vi "取值范围-年月日下拉取值范围.vi"(8 "最小日期":i32[](array[numeric]), 9 "日":refnum<vi>, 10 "月":refnum<vi>, 11 "年":refnum<vi>) -> (0 "错误输出":errorcluster)   [LabVIEW 2017]
uses:
  <vilib>/Utility/miscctls.llb/LVStringsAndValuesArrayTypeDef_U16.ctl
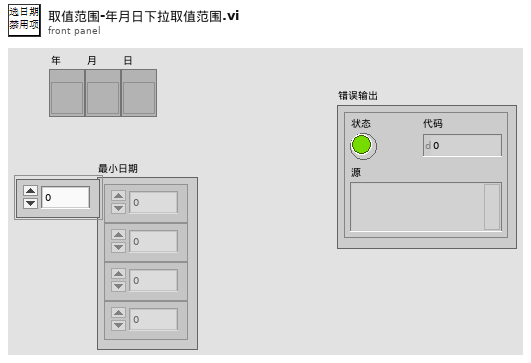
[diagram p1: front panel]
types:
  T1 = typedef "LVStringsAndValuesArrayTypeDef_U16.ctl" = cluster{"String":string, "Value":u16}[]
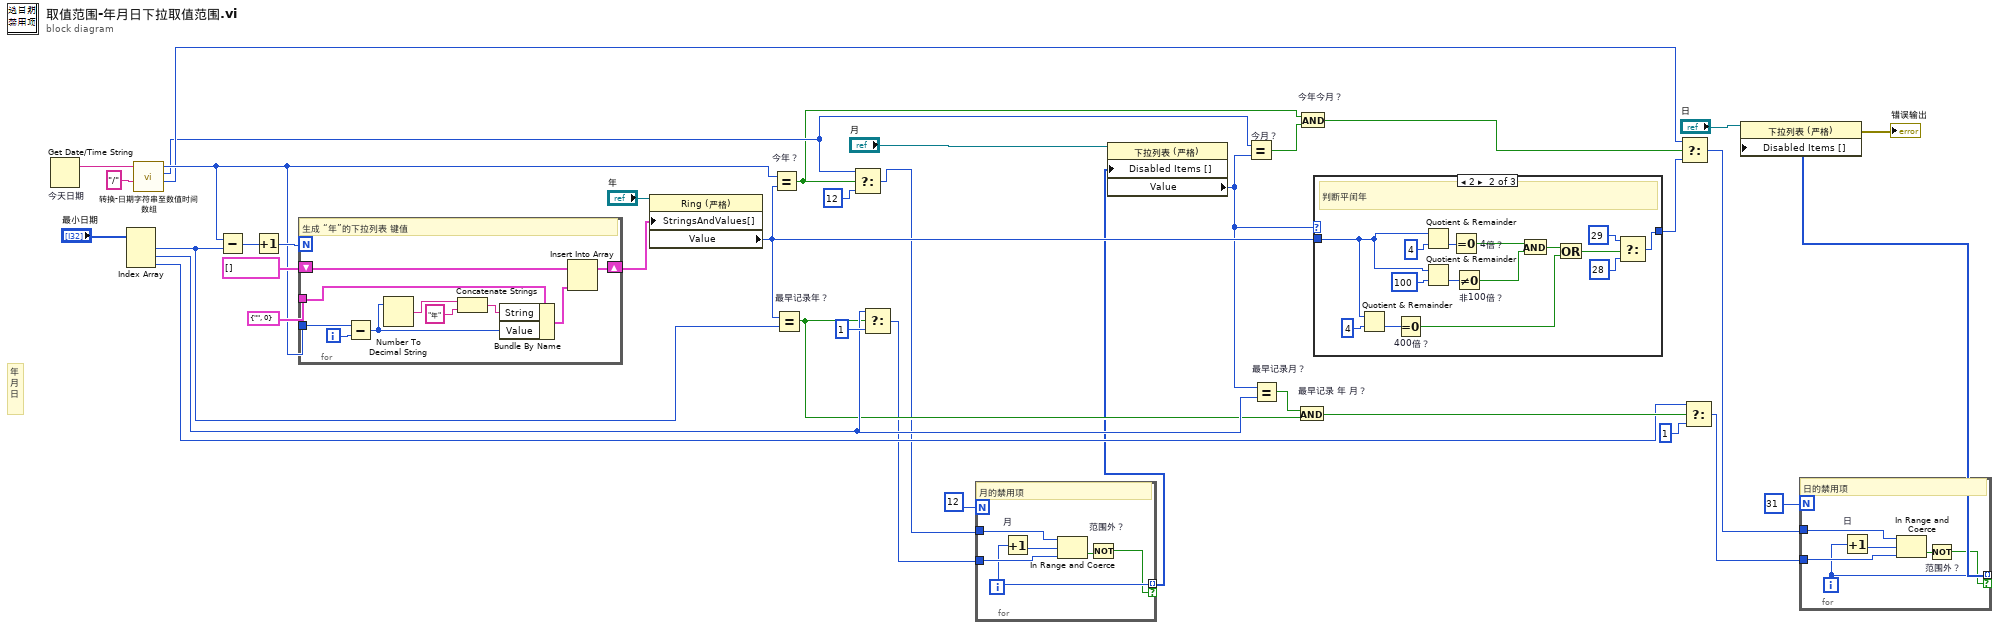
[diagram p0: block diagram]
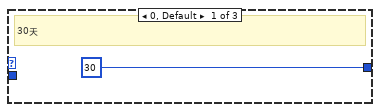
[diagram p2: hidden frame]
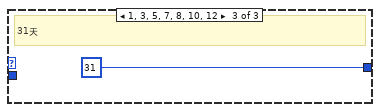
[diagram p3: hidden frame]
diagram:
  # "年\n月\n日"
  n1 = Get Date/Time String "今天日期"() -> (date string=w38:string)  [unwired: 3 in, 1 out]
  n2 = Index Array(array="最小日期") -> (element #1=w21:i32, element #2=w19:i32, element #3=w11:i32)  [unwired: 3 in]
  n3 = call "转换-日期字符串至数值时间数组.vi"("分隔符（/）"="/", "日期时间（或仅日期）字符串"=w38) -> ("D"=w25:i32, "M"=w24:i32, "Y"=w29:i32)  [unwired: 5 in, 2 out]
  n4 = Subtract(x=w29, y=w21) -> (x-y=w34:i32)
  n5 = Increment(x=w34) -> (x+1=w33:i32)
  n6 = for {
    N: w33 -> [_]
    tunnel: w29 -> [w48]
    shift-right: [w43] -> w30
    shift-left: T1 [] ("字符串与值[]") -> [w44]
    tunnel: cluster{"String":string, "Value":u16} {"String"="", "Value"=0} -> [w42]
    i -> [w47]
    # "生成 “年”的下拉列表 键值"
    n7 = Subtract(x=w48, y=w47) -> (x-y=w40:i32)
    n8 = Number To Decimal String(number=w40) -> (decimal integer string=w46:string)  [unwired: 1 in]
    n9 = Concatenate Strings(w46, "年" ("字符串")) -> (w41:string)
    n10 = Bundle By Name(cluster=w42, "String"=w41, "Value"=w40) -> (w39:cluster{"String":string, "Value":u16})
    n11 = Insert Into Array(array=w44, new element=w39) -> (w43:T1)  [unwired: 1 in]
  }
  n12 = property class="Ring (严格)"(reference="年", "StringsAndValues[]"=w30) -> ("Value"=w22:u16)  [unwired: 1 in, 2 out]
  n13 = Equal? "今年？"(x=w29, y=w22) -> (x = y?=w17:bool)
  n14 = Equal? "最早记录年？"(x=w22, y=w21) -> (x = y?=w14:bool)
  n15 = Select(t=w24, s=w17, f=12) -> (s? t:f=w8:i32)
  n16 = Select(t=w19, s=w14, f=1) -> (s? t:f=w7:i32)
  n17 = for {
    N: 12 -> [_]
    tunnel: w8 -> [w54]
    tunnel: w7 -> [w53]
    tunnel: [w51] -> w3 mode=indexing if=w49
    i -> [w51]
    # "月的禁用项"
    n18 = Increment "月"(x=w51) -> (x+1=w52:i32)
    n19 = In Range and Coerce(upper limit=w54, x=w52, lower limit=w53) -> (In Range?=w50:bool)  [unwired: 1 out]
    n20 = Not "范围外？"(x=w50) -> (.not. x?=w49:bool)
  }
  n21 = property class="下拉列表 (严格)"(reference="月", "Disabled Items []"=w3) -> ("Value"=w1:u16)  [unwired: 1 in, 2 out]
  n22 = Equal? "今月？"(x=w24, y=w1) -> (x = y?=w18:bool)
  n23 = Equal? "最早记录月？"(x=w1, y=w19) -> (x = y?=w15:bool)
  n24 = And "最早记录 年 月？"(x=w15, y=w14) -> (x .and. y?=w13:bool)
  n25 = And "今年今月？"(x=w17, y=w18) -> (x .and. y?=w16:bool)
  n26 = case shown="2" w1 {
    tunnel: w22 -> [_ w61 _]
    tunnel: [30 ("f") w65 31 ("f")] -> w23
    frame 0, Default {
      # "30天"
    }
    frame 2 {
      # "判断平闰年"
      n27 = Quotient & Remainder(x=w61, y=u16 4) -> (floor(x/y)=w64:u16)  [unwired: 1 out]
      n28 = Equal To 0? "400倍？"(x=w64) -> (x = 0?=w56:bool)
      n29 = Quotient & Remainder(x=w61, y=u16 4) -> (floor(x/y)=w69:u16)  [unwired: 1 out]
      n30 = Quotient & Remainder(x=w61, y=u16 100) -> (floor(x/y)=w60:u16)  [unwired: 1 out]
      n31 = Equal To 0? "4倍？"(x=w69) -> (x = 0?=w68:bool)
      n32 = Not Equal To 0? "非100倍？"(x=w60) -> (x != 0?=w58:bool)
      n33 = And(x=w68, y=w58) -> (x .and. y?=w59:bool)
      n34 = Or(x=w59, y=w56) -> (x .or. y?=w57:bool)
      n35 = Select(t=29 ("f"), s=w57, f=28) -> (s? t:f=w65:i32)
    }
    frame 1, 3, 5, 7, 8, 10, 12 {
      # "31天"
    }
  }
  n36 = Select(t=w25, s=w16, f=w23) -> (s? t:f=w5:i32)
  n37 = Select(t=w11, s=w13, f=1) -> (s? t:f=w4:i32)
  n38 = for {
    N: 31 -> [_]
    tunnel: w5 -> [w77]
    tunnel: w4 -> [w76]
    tunnel: [w74] -> w2 mode=indexing if=w72
    i -> [w74]
    # "日的禁用项"
    n39 = Increment "日"(x=w74) -> (x+1=w75:i32)
    n40 = In Range and Coerce(upper limit=w77, x=w75, lower limit=w76) -> (In Range?=w73:bool)  [unwired: 1 out]
    n41 = Not "范围外？"(x=w73) -> (.not. x?=w72:bool)
  }
  n42 = property class="下拉列表 (严格)"(reference="日", "Disabled Items []"=w2) -> (error out=→"错误输出":errorcluster)  [unwired: 1 in, 1 out]
